vi "4155C Config Display Y2.vi"(4 "Ymax":dbl format="%.2e", 6 "Ymin":dbl format="%.2e", 8 "error in (no error)":errorcluster, 9 "Logarithmic":bool=TRUE, 10 "SPA Display":bool, 11 "VISA session":refnum<visa-resource-name>) -> (0 "error out":errorcluster, 3 "dup VISA resource name":refnum<visa-resource-name>)   [LabVIEW 2016]
doc: "This VI configures the timing parameters of the measurement functions. The settings of this VI could be different from the actual instrument's settings due to limits imposed by other parameters inside the instrument. To check the actual values of integration time and number of power line cycles, run HP415xA Query Integration Time.vi."
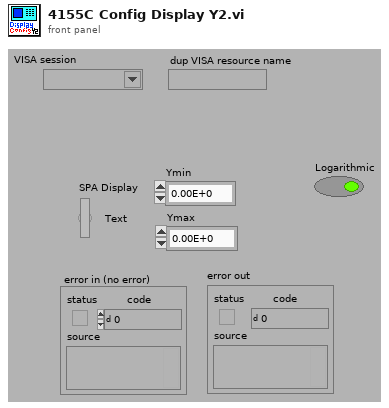
[diagram p1: front panel]
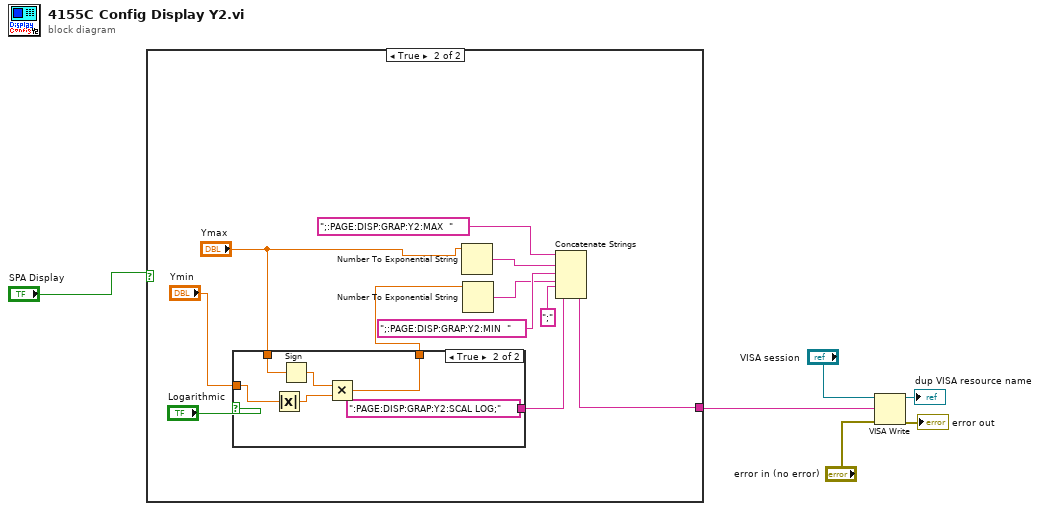
[diagram p0: block diagram]
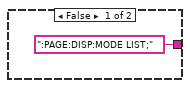
[diagram p2: hidden frame]
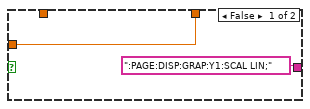
[diagram p3: hidden frame]
diagram:
  n1 = case shown="True" "SPA Display" {
    tunnel: [":PAGE:DISP:MODE LIST;" w11] -> w4
    frame False {
    }
    frame True {
      n2 = case shown="True" "Logarithmic" {
        tunnel: [":PAGE:DISP:GRAP:Y1:SCAL LIN;" ":PAGE:DISP:GRAP:Y2:SCAL LOG;"] -> w12
        tunnel: "Ymax" -> [_ w23]
        tunnel: "Ymin" -> [w19 w22]
        tunnel: [w19 w21] -> w8
        frame False {
        }
        frame True {
          n3 = Absolute Value(x=w22) -> (abs(x)=w25:dbl)
          n4 = Sign(1:w23) -> (0:w24:dbl)
          n5 = Multiply(x=w24, y=w25) -> (x*y=w21:dbl)
        }
      }
      n6 = Number To Exponential String(number="Ymax") -> (E-format string=w15:string)  [unwired: 3 in]
      n7 = Number To Exponential String(number=w8) -> (E-format string=w14:string)  [unwired: 3 in]
      n8 = Concatenate Strings(";:PAGE:DISP:GRAP:Y2:MAX  " ("write buffer (\"\")"), w15, ";:PAGE:DISP:GRAP:Y2:MIN  " ("write buffer (\"\")"), w14, ";" ("Substring"), w12) -> (w11:string)
    }
  }
  n9 = VISA Write(VISA resource name="VISA session", write buffer=w4, error in (no error)="error in (no error)") -> (VISA resource name out=→"dup VISA resource name":refnum<visa-resource-name>, error out=→"error out":errorcluster)  [unwired: 1 out]
